vi "UHR-Fleezers Control (host) - 11.1.vi"() -> ()   [LabVIEW 2012] (continued)
        n2504 = local read "Pump 3 contents"() -> (→"Pump 3 cont disp":string)
      }
      event "Reset Trap Pos. FB": Value Change {
        n2505 = event-data() -> ()  [unwired: 7 out]
        n2506 = xnode "Read/Write Control"("FPGA VI Reference In"=w4152, "error in"=w4151, "Trap Pos. FB Reset"="Reset Trap Pos. FB") -> ()  [unwired: 2 out]
      }
      event "Rem fb disp offset": Value Change {
        n2507 = event-data() -> ()  [unwired: 7 out]
        n2508 = local write "Rem fb disp offset"(FALSE ("Rem fb disp offset")) -> ()
        n2509 = local read "Mean T1 Position (nm)"() -> (w4154:dbl)
        n2510 = local read "FB Trap Pos Offset"() -> (w4155:dbl)
        n2511 = Subtract(x=w4155, y=w4154) -> (x-y=w4153:dbl)
        n2512 = local write "FB Trap Pos Offset"(w4153) -> ()
      }
      event "Threshold (nm)": Value Change {
        n2513 = event-data() -> ()  [unwired: 7 out]
        n2514 = flat-sequence {
          tunnel: w4159 -> [w4167]
          tunnel: w4158 -> [w4166]
          tunnel: [w4160] -> w4157
          tunnel: w4157 -> [w4173]
          frame #0 {
            n2515 = xnode "Read/Write Control"("FPGA VI Reference In"=w4167, "error in"=w4166) -> ("FPGA VI Reference Out"=w4163:T19, "error out"=w4162:errorcluster, "FPGA TTrig Thresh"=w4164:i64)
            n2516 = local read "Threshold stored (nm)"() -> (w4172:dbl)
            n2517 = local read "Threshold (nm)"() -> (w4160:dbl)
            n2518 = local read "AOM X Cal (nm/MHz)"() -> (w4170:dbl)
            n2519 = Subtract(x=w4160, y=w4172) -> (x-y=w4171:dbl)
            n2520 = Divide(x=w4171, y=w4170) -> (x/y=w4168:dbl)
            n2521 = call "IR AOM freq to word.vi"("Frequency In (MHz)"=w4168) -> ("Frequency Word Out (double)"=w4169:dbl)
            n2522 = To Quad Integer(1:w4169) -> (0:w4165:i64)
            n2523 = Add(x=w4164, y=w4165) -> (x+y=w4161:i64)
            n2524 = xnode "Read/Write Control"("FPGA VI Reference In"=w4163, "error in"=w4162, "FPGA TTrig Thresh"=w4161) -> ()  [unwired: 2 out]
          }
          frame #1 {
            "Threshold stored (nm)" <- w4173
          }
        }
      }
      event "FB Trig Integrate": Value Change {
        n2525 = event-data() -> ()  [unwired: 7 out]
        n2526 = local read "FB Trig Integrate"() -> (w4175:u32)
        n2527 = xnode "Read/Write Control"("FPGA VI Reference In"=w4177, "error in"=w4176, "FB Trig Integrate"=w4175) -> ("error out"=w4174:errorcluster)  [unwired: 1 out]
      }
      event "11": Value Change {
        n2528 = event-data() -> ()  [unwired: 7 out]
        n2529 = local read "11"() -> (w4178:bool)
        n2530 = case shown="True" w4178 {
          frame False {
          }
          frame True {
            n2531 = local read "Messages"() -> (w4180:string)
            n2532 = call "Update messages.vi"("Message to add"="You kicked it up to 11!", "Old message string"=w4180) -> ("New message string"=w4181:string)
            n2533 = call <vilib>:"Beep.vi"() -> ()  [unwired: 12 in]
            n2534 = local write "Messages"(w4181) -> ()
          }
        }
      }
      event "Trap Pos. FB ON": Value Change {
        n2535 = event-data() -> ()  [unwired: 7 out]
        n2536 = xnode "Read/Write Control"("FPGA VI Reference In"=w4184, "error in"=w4183, "Force feedback"="Trap Pos. FB ON") -> ()  [unwired: 2 out]
      }
      event "Remove Action Offset": Value Change {
        n2537 = event-data() -> ()  [unwired: 7 out]
        n2538 = local write "Remove Action Offset"(FALSE ("Remove Action Offset")) -> ()
        n2539 = local read "Trap Pos. FB Mult Factor"() -> (w4189:i64)
        n2540 = local read "Trap Pos FB Action"() -> (w4187:i64)
        n2541 = local read "Trap Pos. FB Offset Factor"() -> (w4185:i64)
        n2542 = Multiply(x=w4189, y=w4187) -> (x*y=w4188:i64)
        n2543 = Add(x=w4188, y=w4185) -> (x+y=w4186:i64)
        n2544 = local write "Trap Pos. FB Offset Factor"(w4186) -> ()
        n2545 = xnode "Read/Write Control"("FPGA VI Reference In"=w4192, "error in"=w4191, "Trap Pos. FB Offset Factor"=w4186) -> ()  [unwired: 2 out]
      }
      event "Remove Unwinding Offset": Value Change {
        n2546 = event-data() -> ()  [unwired: 7 out]
        n2547 = local write "Remove Unwinding Offset"(FALSE ("Remove Action Offset")) -> ()
        n2548 = local read "Trap Pos. FB Mult Factor"() -> (w4204:i64)
        n2549 = local read "Trap Pos FB Action"() -> (w4202:i64)
        n2550 = local read "Trap Pos. FB Offset Factor"() -> (w4201:i64)
        n2551 = Multiply(x=w4204, y=w4202) -> (x*y=w4203:i64)
        n2552 = local read "Trap Pos. FB Mult Factor"() -> (w4200:i64)
        n2553 = Add(x=w4203, y=w4201) -> (x+y=w4194:i64)
        n2554 = Multiply(x=32768, y="factor") -> (x*y=w4197:dbl)
        n2555 = Multiply(x=w4197, y=w4200) -> (x*y=w4199:dbl)
        n2556 = Subtract(x=w4194, y=w4199) -> (x-y=w4198:dbl)
        n2557 = To Quad Integer(1:w4198) -> (0:w4193:i64)
        n2558 = xnode "Read/Write Control"("FPGA VI Reference In"=w4207, "error in"=w4206, "Trap Pos. FB Offset Factor"=w4193) -> ()  [unwired: 2 out]
        n2559 = local write "Trap Pos. FB Offset Factor"(w4193) -> ()
      }
      event "Trap Pos. FB Range", "Trap Pos. FB Gains", "Trap Pos. FB Mult Factor", "Trap Pos. FB Offset Factor", "Trap Pos FB Negate Action", "Trap Pos FB Monitor\nT1 or T2", "Differential FB?", "Negate Diff?": Value Change {
        n2560 = event-data() -> ()  [unwired: 7 out]
        n2561 = local read "Negate Diff?"() -> (w4208:bool)
        n2562 = xnode "Read/Write Control"("FPGA VI Reference In"=w4218, "error in"=w4217, "Trap Pos. FB Range"="Trap Pos. FB Range", "Trap Pos. FB Gains"="Trap Pos. FB Gains", "Trap Pos. FB Mult Factor"="Trap Pos. FB Mult Factor", "Trap Pos. FB Offset Factor"="Trap Pos. FB Offset Factor", "Trap Pos FB Negate Action"="Trap Pos FB Negate Action", "Trap Pos FB Monitor T1 or T2"="Trap Pos FB Monitor\nT1 or T2", "AI1 X Scale"="Trap Pos. AI1 X Pre-scale", "Negate Diff?"=w4208, "Diff FB Measurement?"="Differential FB?") -> ()  [unwired: 2 out]
      }
      event "Trap Pos FB SP", "Trap Pos FB SP 2", "Use SP 2": Value Change {
        n2563 = event-data() -> ()  [unwired: 7 out]
        n2564 = Select(t="Trap Pos FB SP 2", s="Use SP 2", f="Trap Pos FB SP") -> (s? t:f=w4219:fxp<+/-,16,1>)
        n2565 = xnode "Read/Write Control"("FPGA VI Reference In"=w4224, "error in"=w4223, "Trap Pos. FB SP"=w4219) -> ()  [unwired: 2 out]
      }
      event "Offset SP2 from SP1": Value Change {
        n2566 = event-data() -> ()  [unwired: 7 out]
        n2567 = local read "Trap Pos FB SP"() -> (w4227:fxp<+/-,16,1>)
        n2568 = Add(x=w4227, y="SP2 Offset") -> (x+y=w4225:fxp<+/-,16,1>)
        n2569 = property on="Trap Pos FB SP 2" class="DigNum (strict)"("Val(Sgnl)"=w4225) -> ()  [unwired: 2 in, 2 out]
        n2570 = local write "Offset SP2 from SP1"(FALSE ("Offset SP2 from SP1")) -> ()
      }
      event "Set Reading to\nSetpoint": Value Change {
        # "This is the actual PID input signal"
        n2571 = event-data() -> ()  [unwired: 7 out]
        n2572 = local write "Set Reading to\nSetpoint"(FALSE ("Set SP to Reading")) -> ()
        n2573 = xnode "Read/Write Control"("FPGA VI Reference In"=w4233, "error in"=w4232) -> ("FPGA VI Reference Out"=w4231:T19, "error out"=w4230:errorcluster, "Trap Pos FB Int-Norm Signal"=w4229:fxp<+/-,16,1>)
        n2574 = local read "Differential FB?"() -> (w4234:bool)
        n2575 = case shown="False" w4234 {
          tunnel: [w4239 w4246] -> w4236
          tunnel: w4229 -> [w4237 w4246]
          frame False {
            n2576 = local read "Trap Pos FB Monitor\nT1 or T2"() -> (w4242:bool)
            n2577 = local read "Trap X AI1 (DMA)"() -> (w4245:T13)
            n2578 = Unbundle By Name(w4245) -> ("Set 1"=w4244:fxp<+/-,16,1>, "Set 2"=w4243:fxp<+/-,16,1>)
            n2579 = Select(t=w4244, s=w4242, f=w4243) -> (s? t:f=w4241:fxp<+/-,16,1>)
            n2580 = Not(x="Set SP Using...") -> (.not. x?=w4238:bool)
            n2581 = Select(t=w4237, s=w4238, f=w4241) -> (s? t:f=w4239:fxp<+/-,16,1>)
          }
          frame True {
          }
        }
        n2582 = xnode "Read/Write Control"("FPGA VI Reference In"=w4231, "error in"=w4230, "Trap Pos. FB SP"=w4236) -> ()  [unwired: 2 out]
        n2583 = local write "Trap Pos FB SP"(w4236) -> ()
      }
      event "Trap Pos. FB Out Scale 2^n": Value Change {
        n2584 = event-data() -> ()  [unwired: 7 out]
        n2585 = Scale By Power Of 2(n="Trap Pos. FB Out Scale 2^n", x=ext 1.0) -> (x*2^n=w4247:ext)
        n2586 = property on="Trap Pos. FB Mult Factor" class="DigNum (strict)"("Val(Sgnl)"=w4247) -> ()  [unwired: 2 in, 2 out]
      }
      event "Trap Pos FB Int Count": Value Change {
        n2587 = event-data() -> ()  [unwired: 7 out]
        n2588 = xnode "Read/Write Control"("FPGA VI Reference In"=w4252, "error in"=w4251, "Trap Pos FB Int Count"="Trap Pos FB Int Count") -> ()  [unwired: 2 out]
      }
      event "Trap pos": Value Change {
        n2589 = event-data() -> ()  [unwired: 7 out]
        n2590 = case shown="True" "Trap pos" {
          frame False {
            n2591 = property on="Trap Delta Graph" class="WFGraph (strict)"("Visible"=TRUE) -> ()  [unwired: 2 in, 2 out]
            n2592 = property on="Saved trap pos" class="WFGraph (strict)"("Visible"=FALSE) -> ()  [unwired: 2 in, 2 out]
          }
          frame True {
            n2593 = property on="Saved trap pos" class="WFGraph (strict)"("Visible"=TRUE) -> ()  [unwired: 2 in, 2 out]
            n2594 = property on="Trap Delta Graph" class="WFGraph (strict)"("Visible"=FALSE) -> ()  [unwired: 2 in, 2 out]
          }
        }
      }
    }
    "error out 2" <- w3157
    n2595 = node-c288() -> ()  [unwired: 2 out]
  }
  n2596 = timed-loop "Oscillate Trap/AOM (fishing, debugging)" {
    tunnel: w6 -> [w4259]
    tunnel: [w4258] -> w100
    timing: w95 -> [_]
    timing-out: [_] -> w94
    stop <- w4258 stop-if-true
    n2597 = node-c288() -> ()  [unwired: 2 out]
    n2598 = event shown="[0] \"Oscillate Set 1\", \"Fish for Tether\": Value Change" {
      selector: _ -> [_ _ _]
      dyn-events: _ -> [_ _ _]
      timeout: _ -> [_ _ _]
      tunnel: w4259 -> [w4266 _ _]
      tunnel: [FALSE ("Stop All") _ w4855] -> w4258
      event "Oscillate Set 1", "Fish for Tether": Value Change {
        n2599 = event-data() -> ()  [unwired: 6 out]
        n2600 = local read "Oscillate Set 1"() -> (w4265:bool)
        n2601 = Or(x=w4265, y="Fish for Tether") -> (x .or. y?=w4263:bool)
        n2602 = case shown="True" w4263 {
          tunnel: w4266 -> [_ w4269]
          tunnel: "Fish for Tether" -> [_ w4268]
          frame False {
          }
          frame True {
            n2603 = case shown="True" w4268 {
              selector: w4268 -> [w4272 w4278]
              tunnel: [w4272 w4278] -> w4267
              frame False {
              }
              frame True {
                n2604 = local write "Scan axis 2"(TRUE) -> ()
                n2605 = local write "Tether"(FALSE ("Tether")) -> ()
                n2606 = local read "Flow ON during cal?"() -> (w4273:bool)
                n2607 = property on="Trap Delta (MHz)" class="DigNum (strict)"("Val(Sgnl)"="Furthest Delta (MHz)") -> ()  [unwired: 2 in, 2 out]
                n2608 = Or(x="Flow ON during \nfishing?", y=w4273) -> (x .or. y?=w4274:bool)
                n2609 = Wait (ms)(milliseconds to wait=u32 500) -> ()  [unwired: 1 out]
                n2610 = property on="Sample Channel\nFlow" class="Bool (strict)"("Val(Sgnl)"=w4274) -> ()  [unwired: 2 in, 2 out]
              }
            }
            n2611 = node-c288() -> (w4271:T21)  [unwired: 4 out]
            n2612 = timed-loop "Oscillate AOD" {
              timing: w4271 -> [_]
              timing-out: [_] -> w4270
              tunnel: w4269 -> [w4288]
              tunnel: w4267 -> [w4281]
              i -> [w4290]
              stop <- w4287 stop-if-true
              n2613 = node-c288() -> (w4289:i64)  [unwired: 1 out]
              n2614 = flat-sequence {
                tunnel: w4290 -> [w4317]
                tunnel: w4289 -> [w4316]
                tunnel: w4288 -> [w4295]
                tunnel: w4281 -> [w4298]
                tunnel: [w4298] -> w4286
                tunnel: [w4297] -> w4285
                tunnel: [w4294] -> w4284
                tunnel: [w4291] -> w4282
                tunnel: w4286 -> [w4353]
                tunnel: w4285 -> [w4351]
                tunnel: w4284 -> [w4350]
                tunnel: [w4349] -> w4283
                tunnel: w4282 -> [w4348]
                tunnel: [w4425] -> w4287
                tunnel: w4283 -> [w4424]
                frame #0 {
                  n2615 = Divide(x=w4316, y=i64 1000) -> (x/y=w4311:dbl)
                  n2616 = Multiply(x=w4311, y=w4317) -> (x*y=w4313:dbl)
                  n2617 = local read "BD 1 Frequency 2 (MHz)"() -> (w4296:dbl)
                  n2618 = Multiply(x="Osc. freq. (Hz)", y=6.283185307179586) -> (x*y=w4314:dbl)
                  n2619 = Multiply(x=w4314, y=w4313) -> (x*y=w4293:dbl)
                  n2620 = local read "BD 1 Frequency 1 (MHz)"() -> (w4301:dbl)
                  n2621 = local read "BD 2 Frequency 1 (MHz)"() -> (w4300:dbl)
                  n2622 = case shown="True" w4298 {
                    tunnel: w4293 -> [w4323 w4328]
                    tunnel: w4301 -> [_ w4339]
                    tunnel: w4296 -> [_ w4340]
                    tunnel: [w4320 w4334] -> w4299
                    tunnel: [FALSE w4331] -> w4294
                    tunnel: [0.0 w4324] -> w4291
                    frame False {
                      n2623 = Sine(x=w4323) -> (sin(x)=w4321:dbl)
                      n2624 = Multiply(x=w4321, y="Osc. amp. (MHz)") -> (x*y=w4320:dbl)
                    }
                    frame True {
                      n2625 = Cosine(x=w4328) -> (cos(x)=w4343:dbl)
                      n2626 = Subtract(x=w4340, y=w4339) -> (x-y=w4338:dbl)
                      n2627 = Decrement(x=w4343) -> (x-1=w4342:dbl)
                      n2628 = Subtract(x=w4338, y="Closest Delta (MHz)") -> (x-y=w4335:dbl)
                      n2629 = Divide(x=w4342, y=-2.0) -> (x/y=w4336:dbl)
                      n2630 = Multiply(x=w4336, y=w4335) -> (x*y=w4334:dbl)
                      n2631 = local read "Vec Mean of T1 T2"() -> (w4330:dbl[])
                      n2632 = Greater?(x=w4330, y="Stop F (pN)") -> (0:w4332:bool[])
                      n2633 = Or Array Elements(Boolean array=w4332) -> (logical OR=w4331:bool)
                      n2634 = Divide(x=w4328, y=6.283185307179586) -> (x/y=w4327:dbl)
                      n2635 = Round Toward +Infinity(x=w4327) -> (ceil(x): smallest int >= x=w4324:dbl)
                      "Attempts" <- w4324
                      n2636 = Greater?(x=w4324, y="Attempt Limit") -> (0:w4326:bool)
                      n2637 = case shown="True" w4326 {
                        frame False {
                        }
                        frame True {
                          n2638 = local write "Fish for Tether"(FALSE ("Fish for Tether")) -> ()
                          n2639 = call <vilib>:"Beep.vi"() -> ()  [unwired: 3 in, 9 out]
                          n2640 = local read "Messages"() -> (w4345:string)
                          n2641 = call "Update messages.vi"("Message to add"="Tether fishing timeout." ("Messages"), "Old message string"=w4345) -> ("New message string"=→"Messages":string)
                        }
                      }
                    }
                  }
                  n2642 = Select(t=w4301, s="Scan axis 2", f=w4300) -> (s? t:f=w4304:dbl)
                  n2643 = Add(x=w4299, y=w4304) -> (x+y=w4297:dbl)
                  n2644 = Select(t=w4297, s="Scan axis 2", f=w4301) -> (s? t:f=w4307:dbl)
                  n2645 = Select(t=w4300, s="Scan axis 2", f=w4297) -> (s? t:f=w4306:dbl)
                  n2646 = local read "Y RF Frequency Limits (MHz)"() -> (w4302:T16)
                  n2647 = local read "X RF Frequency Limits (MHz)"() -> (w4303:T16)
                  n2648 = local read "BD 1 Frequency 3 (MHz)"() -> (w4310:dbl)
                  n2649 = local read "BD 2 Frequency 2 (MHz)"() -> (w4309:dbl)
                  n2650 = local read "BD 2 Frequency 3 (MHz)"() -> (w4308:dbl)
                  n2651 = call "set RF board frequency - interlace.vi"("Board 2 Frequency Limits"=w4302, "Board 1 Frequency Limits"=w4303, "FPGA VI Reference In"=w4295, "Board 2 Frequency 3 (MHz)"=w4308, "Board 1 Frequency 3 (MHz)"=w4310, "Board 2 Frequency 2 (MHz)"=w4309, "Board 2 Frequency 1 (MHz)"=w4306, "Board 1 Frequency 2 (MHz)"=w4296, "Board 1 Frequency 1  (MHz)"=w4307) -> ()  [unwired: 1 in, 2 out]
                }
                frame #1 {
                  n2652 = And(x=w4353, y=w4350) -> (x .and. y?=w4352:bool)
                  n2653 = case "Only if were fishing and now formed tether" shown="False" w4352 {
                    tunnel: w4351 -> [w4355 w4370]
                    tunnel: [w4354 w4369] -> w4349
                    tunnel: w4348 -> [_ w4365]
                    frame False {
                      n2654 = local read "Fish for Tether"() -> (w4354:bool)
                      n2655 = case shown="False" w4354 {
                        tunnel: w4355 -> [w4356 _]
                        frame False {
                          n2656 = property on="BD 1 Frequency 1 (MHz)" class="DigNum (strict)"("Val(Sgnl)"=w4356) -> ()  [unwired: 2 in, 2 out]
                        }
                        frame True {
                        }
                      }
                    }
                    frame True {
                      w4369 = FALSE ("Fish for Tether")
                      n2657 = call <vilib>:"Beep.vi"() -> ()  [unwired: 3 in, 9 out]
                      n2658 = Number To Decimal String(number=w4365, width (-)=i16 1) -> (decimal integer string=w4363:string)
                      n2659 = Concatenate Strings("Formed tether in ", w4363, " attempt(s)." ("string")) -> (w4360:string)
                      n2660 = local read "Messages"() -> (w4367:string)
                      n2661 = local write "Fish for Tether"(w4369) -> ()
                      n2662 = call "Update messages.vi"("Message to add"=w4360, "Old message string"=w4367) -> ("New message string"=w4366:string)
                      n2663 = local write "Messages"(w4366) -> ()
                      n2664 = Get Date/Time In Seconds() -> (seconds since 1Jan1904=→"Time tether formed":timestamp)
                      n2665 = local read "Flow ON during cal?"() -> (w4357:bool)
                      n2666 = property on="Sample Channel\nFlow" class="Bool (strict)"("Val(Sgnl)"=w4357) -> (error out=w4358:errorcluster)  [unwired: 2 in, 1 out]
                      n2667 = case shown="\"2\", \"3\", \"4\", \"5\", \"6\"" "Then..." {
                        selector: "Then..." -> [_ w4373]
                        tunnel: w4370 -> [w4372 _]
                        tunnel: w4358 -> [_ _]
                        frame "1", Default {
                          n2668 = property on="BD 1 Frequency 1 (MHz)" class="DigNum (strict)"("Val(Sgnl)"=w4372) -> ()  [unwired: 2 in, 2 out]
                        }
                        frame "2", "3", "4", "5", "6" {
                          n2669 = flat-sequence {
                            tunnel: w4373 -> [w4375]
                            frame #0 {
                              n2670 = property on="Trap Delta (MHz)" class="DigNum (strict)"("Val(Sgnl)"="Move to Delta 1 (MHz)") -> ()  [unwired: 2 in, 2 out]
                            }
                            frame #1 {
                              n2671 = case shown="\"5\", \"6\"" w4375 {
                                selector: w4375 -> [w4378 w4388 _]
                                frame "3", "4" {
                                n2672 = flat-sequence {
                                tunnel: w4378 -> [w4379]
                                tunnel: [w4379] -> w4376
                                tunnel: [w4381] -> w4377
                                tunnel: w4376 -> [w4381]
                                tunnel: w4377 -> [w4385]
                                frame #0 {
                                n2673 = property on="Green Laser ON/Interlacing" class="Bool (strict)"("Val(Sgnl)"=TRUE ("Value (Signaling)")) -> ()  [unwired: 2 in, 2 out]
                                }
                                frame #1 {
                                n2674 = Multiply(x="Wait Before Save (s)", y=u32 1000 ("x")) -> (x*y=w4383:u32)
                                n2675 = Wait (ms)(milliseconds to wait=w4383) -> ()  [unwired: 1 out]
                                }
                                frame #2 {
                                n2676 = property on="Start Saving" class="Bool (strict)"("Value"=TRUE ("Start Saving")) -> ()  [unwired: 2 in, 2 out]
                                n2677 = case shown="\"4\"" w4385 {
                                frame Default {
                                }
                                frame "4" {
                                n2678 = property on="Fl. Triggered..." class="Bool (strict)"("Val(Sgnl)"=TRUE ("Value (Signaling)")) -> ()  [unwired: 2 in, 2 out]
                                }
                                }
                                }
                                }
                                }
                                frame "5", "6" {
                                n2679 = stacked-sequence {
                                tunnel: w4388 -> [_ _ _ _ _ _ w4400]
                                frame #0 {
                                n2680 = Replace Array Subset(array=u32[] [0] ("Index Values"), new element="Raster Set Upon Tether", index=0) -> (w4389:u32[])
                                n2681 = property on="Saved AOD Raster Scan Parameter Sets" class="Arr (strict)"("Index Values"=w4389) -> ()  [unwired: 2 in, 2 out]
                                }
                                frame #1 {
                                n2682 = Wait (ms)(milliseconds to wait=u32 500) -> ()  [unwired: 1 out]
                                }
                                frame #2 {
                                n2683 = property on="Load parameters" class="Bool (strict)"("Val(Sgnl)"=TRUE ("Value (Signaling)")) -> ()  [unwired: 2 in, 2 out]
                                n2684 = case shown="True" "Green ON During Raster" {
                                frame False {
                                }
                                frame True {
                                n2685 = property on="Green Laser ON/Interlacing" class="Bool (strict)"("Val(Sgnl)"=TRUE ("Value (Signaling)")) -> ()  [unwired: 2 in, 2 out]
                                }
                                }
                                }
                                frame #3 {
                                n2686 = Wait (ms)(milliseconds to wait=u32 500) -> ()  [unwired: 1 out]
                                }
                                frame #4 {
                                n2687 = property on="Trap Raster Scan" class="Bool (strict)"("Val(Sgnl)"=TRUE ("Value (Signaling)")) -> ()  [unwired: 2 in, 2 out]
                                }
                                frame #5 {
                                n2688 = Wait (ms)(milliseconds to wait=u32 2000) -> ()  [unwired: 1 out]
                                }
                                frame #6 {
                                n2689 = flat-sequence {
                                tunnel: w4400 -> [w4407]
                                frame #0 {
                                n2690 = while {
                                stop <- w4403 stop-if-true
                                n2691 = local read "Raster Scanning..."() -> (w4402:bool)
                                n2692 = local read "Saving..."() -> (w4405:bool)
                                n2693 = Wait (ms)(milliseconds to wait=u32 100) -> ()  [unwired: 1 out]
                                n2694 = Not(x=w4405) -> (.not. x?=w4404:bool)
                                n2695 = Not(x=w4402) -> (.not. x?=w4401:bool)
                                n2696 = And(x=w4404, y=w4401) -> (x .and. y?=w4403:bool)
                                }
                                }
                                frame #1 {
                                n2697 = local read "Tether"() -> (w4408:bool)
                                n2698 = case shown="True" w4408 {
                                tunnel: w4407 -> [_ w4410]
                                frame False {
                                n2699 = property on="Fish for Tether" class="Bool (strict)"("Val(Sgnl)"="Fish again after \nraster break?") -> ()  [unwired: 2 in, 2 out]
                                }
                                frame True {
                                n2700 = stacked-sequence {
                                tunnel: w4410 -> [_ w4414 _ _]
                                frame #0 {
                                n2701 = property on="Trap Delta (MHz)" class="DigNum (strict)"("Val(Sgnl)"="Move to Delta 2 (MHz)") -> ()  [unwired: 2 in, 2 out]
                                n2702 = case shown="True" "Flow ON after\ntether testing?" {
                                frame False {
                                }
                                frame True {
                                n2703 = property on="Sample Channel\nFlow" class="Bool (strict)"("Val(Sgnl)"=TRUE ("Value (Signaling)")) -> ()  [unwired: 2 in, 2 out]
                                }
                                }
                                }
                                frame #1 {
                                n2704 = flat-sequence {
                                tunnel: w4414 -> [w4416]
                                frame #0 {
                                n2705 = Wait (ms)(milliseconds to wait=u32 500) -> ()  [unwired: 1 out]
                                }
                                frame #1 {
                                n2706 = case shown="\"6\"" w4416 {
                                frame Default {
                                }
                                frame "6" {
                                n2707 = property on="Green Laser ON/Interlacing" class="Bool (strict)"("Val(Sgnl)"=TRUE ("Green Laser ON/Interlacing")) -> ()  [unwired: 2 in, 2 out]
                                }
                                }
                                }
                                frame #2 {
                                n2708 = Wait (ms)(milliseconds to wait=u32 500) -> ()  [unwired: 1 out]
                                }
                                frame #3 {
                                n2709 = local write "Start Saving"("Save at end (5, 6)") -> ()
                                }
                                }
                                }
                                frame #2 {
                                n2710 = local read "Bead Sep. Int. Time (s)"() -> (w4422:dbl)
                                n2711 = Multiply(x=w4422, y=1000.0) -> (x*y=w4421:dbl)
                                n2712 = Wait (ms)(milliseconds to wait=w4421) -> ()  [unwired: 1 out]
                                }
                                frame #3 {
                                n2713 = property on="Remove Offset" class="Bool (strict)"("Val(Sgnl)"=TRUE ("Value (Signaling)")) -> ()  [unwired: 2 in, 2 out]
                                }
                                }
                                }
                                }
                                }
                                }
                                }
                                }
                                }
                                frame "2", Default {
                                }
                              }
                            }
                          }
                        }
                      }
                      "Tether" <- "Tether Alarm?"
                    }
                  }
                }
                frame #2 {
                  n2714 = local read "Oscillate Set 1"() -> (w4429:bool)
                  n2715 = local read "Stop All"() -> (w4427:bool)
                  n2716 = Or(x=w4429, y=w4424) -> (x .or. y?=w4426:bool)
                  n2717 = Not(x=w4426) -> (.not. x?=w4428:bool)
                  n2718 = Compound Arithmetic op=OR(w4427, w4428) -> (w4425:bool)
                }
              }
              n2719 = node-c288() -> ()  [unwired: 2 out]
            }
            n2720 = node-c288(w4270) -> ()  [unwired: 1 out]
          }
        }
      }
      event "Fl. Triggered...": Value Change {
        n2721 = event-data() -> ()  [unwired: 7 out]
        n2722 = case shown="True" "Fl. Triggered..." {
          frame False {
          }
          frame True {
            n2723 = node-c288() -> (w4440:T21)  [unwired: 4 out]
            n2724 = timed-loop {
              timing: w4440 -> [_]
              timing-out: [_] -> w4439
              tunnel: "Action" -> [w4448]
              shift-right: [w4445] -> _
              shift-left: u8 255 -> [w4447]
              shift-right: [w4442] -> _
              shift-left: 255 -> [w4444]
              stop <- w4441 stop-if-true
              # "Reset confocal spot"
              n2725 = node-c288() -> ()  [unwired: 2 out]
              n2726 = flat-sequence {
                tunnel: w4448 -> [w4468]
                tunnel: w4447 -> [w4467]
                tunnel: [w4466] -> w4446
                tunnel: w4444 -> [w4453]
                tunnel: [w4452] -> w4443
                tunnel: [w4847] -> w4441
                tunnel: w4446 -> [w4846]
                tunnel: [w4846] -> w4445
                tunnel: [w4845] -> w4442
                tunnel: w4443 -> [w4845]
                frame #0 {
                  n2727 = local read "Delta Fl. 2"() -> (w4465:dbl)
                  n2728 = local read "Delta Fl. 1"() -> (w4460:dbl)
                  n2729 = Multiply(x="Fl. Delta Thresh. (kHz)", y=1000.0) -> (x*y=w4455:dbl)
                  n2730 = Select(t=w4460, s="APD to Watch", f=w4465) -> (s? t:f=w4456:dbl)
                  n2731 = Greater?(x=w4456, y=w4455) -> (0:w4461:bool)
                  n2732 = Or(x="Force Yank", y=w4461) -> (x .or. y?=w4459:bool)
                  n2733 = And(x=w4459, y="Yank when?") -> (x .and. y?=w4457:bool)
                  n2734 = case shown="False" w4457 {
                    tunnel: w4468 -> [w4471 w4672]
                    tunnel: w4467 -> [w4473 w4668]
                    tunnel: [w4473 w4666] -> w4466
                    tunnel: w4456 -> [w4479 _]
                    tunnel: w4455 -> [w4478 _]
                    tunnel: "Force Yank" -> [w4476 _]
                    tunnel: w4453 -> [w4475 w4665]
                    tunnel: [w4474 w4665] -> w4452
                    frame False {
                      n2735 = Negate(x=w4478) -> (-x=w4470:dbl)
                      n2736 = local write "Fl. High"(TRUE ("Fl. High")) -> ()
                      n2737 = Less?(x=w4479, y=w4470) -> (x < y?=w4477:bool)
                      n2738 = Or(x=w4476, y=w4477) -> (x .or. y?=w4472:bool)
                      n2739 = case shown="True" w4472 {
                        tunnel: w4475 -> [w4480 w4490]
                        tunnel: [w4480 w4489] -> w4474
                        tunnel: w4471 -> [_ w4488]
                        frame False {
                        }
                        frame True {
                          n2740 = flat-sequence {
                            tunnel: w4490 -> [w4496]
                            tunnel: w4488 -> [w4493]
                            tunnel: [w4495] -> w4487
                            tunnel: [w4494] -> w4486
                            tunnel: [w4493] -> w4485
                            tunnel: w4484 -> [w4492]
                            tunnel: [w4492] -> w4483
                            tunnel: w4482 -> [w4491]
                            tunnel: [w4491] -> w4481
                            tunnel: [w4567] -> w4489
                            tunnel: w4487 -> [w4567]
                            tunnel: w4486 -> [w4566]
                            tunnel: w4485 -> [w4565]
                            tunnel: w4483 -> [w4564]
                            tunnel: w4481 -> [w4563]
                            frame #0 {
                              n2741 = call <vilib>:"Beep.vi"() -> ()  [unwired: 12 in]
                              n2742 = local write "Waiting"(FALSE ("Waiting")) -> ()
                              n2743 = Increment(x=w4496) -> (x+1=w4495:i32)
                              n2744 = case shown="\"Yank\"" w4493 {
                                tunnel: w4495 -> [_ w4501 _]
                                frame "Alarm", Default {
                                }
                                frame "Yank" {
                                n2745 = flat-sequence {
                                tunnel: w4501 -> [w4504]
                                tunnel: [w4503] -> w4500
                                tunnel: [w4502] -> w4499
                                tunnel: w4500 -> [w4514]
                                tunnel: w4499 -> [w4515]
                                frame #0 {
                                n2746 = local read "Yank Delay (s)"() -> (w4507:dbl)
                                n2747 = local read "N Array El"() -> (w4502:u8)
                                n2748 = Quotient & Remainder(x=w4504, y=w4502) -> (x-y*floor(x/y)=w4503:i32)  [unwired: 1 out]
                                n2749 = Multiply(x=w4507, y=1000.0) -> (x*y=w4505:dbl)
                                n2750 = Wait (ms)(milliseconds to wait=w4505) -> ()  [unwired: 1 out]
                                }
                                frame #1 {
                                n2751 = local read "Yank to which?"() -> (w4509:bool)
                                n2752 = local read "Random Choice"() -> (w4519:bool)
                                n2753 = local read "Yank to Trap Delta (MHz)"() -> (w4512:dbl[])
                                n2754 = local read "Yank to SP"() -> (w4513:dbl[])
                                n2755 = Random Number (0-1)() -> (number: 0 to 1=w4518:dbl)
                                n2756 = Multiply(x=w4515, y=w4518) -> (x*y=w4517:dbl)
                                n2757 = Round Toward -Infinity(1:w4517) -> (0:w4516:dbl)
                                n2758 = Select(t=w4516, s=w4519, f=w4514) -> (s? t:f=w4510:dbl)
                                n2759 = Select(t=w4512, s=w4509, f=w4513) -> (s? t:f=w4511:dbl[])
                                n2760 = Index Array(array=w4511, index=w4510) -> (element=w4508:dbl)
                                n2761 = case shown="True" w4509 {
                                tunnel: w4508 -> [w4520 w4547]
                                frame False {
                                n2762 = flat-sequence {
                                tunnel: w4520 -> [w4521]
                                frame #0 {
                                n2763 = property on="Trap Pos FB SP" class="DigNum (strict)"("Val(Sgnl)"=w4521) -> ()  [unwired: 2 in, 2 out]
                                }
                                frame #1 {
                                n2764 = Wait (ms)(milliseconds to wait=u32 700) -> ()  [unwired: 1 out]
                                }
                                frame #2 {
                                n2765 = local read "Action (%)"() -> (w4526:dbl)
                                n2766 = Absolute Value(x=w4526) -> (abs(x)=w4525:dbl)
                                n2767 = Greater?(x=w4525, y=70.0) -> (0:w4523:bool)
                                n2768 = property on="Remove Action Offset" class="Bool (strict)"("Val(Sgnl)"=w4523) -> ()  [unwired: 2 in, 2 out]
                                }
                                frame #3 {
                                n2769 = for {
                                N: 4 -> [_]
                                n2770 = flat-sequence {
                                frame #0 {
                                n2771 = Wait (ms)(milliseconds to wait=u32 500) -> ()  [unwired: 1 out]
                                }
                                frame #1 {
                                n2772 = local read "Action (%)"() -> (w4532:dbl)
                                n2773 = Absolute Value(x=w4532) -> (abs(x)=w4531:dbl)
                                n2774 = Greater?(x=w4531, y=70.0) -> (0:w4529:bool)
                                n2775 = property on="Remove Action Offset" class="Bool (strict)"("Val(Sgnl)"=w4529) -> ()  [unwired: 2 in, 2 out]
                                }
                                }
                                }
                                }
                                frame #4 {
                                n2776 = Wait (ms)(milliseconds to wait=u32 500) -> ()  [unwired: 1 out]
                                }
                                frame #5 {
                                n2777 = local read "Mean"() -> (w4540:dbl)
                                n2778 = Greater?(x=w4540, y=11.0) -> (0:w4534:bool)
                                n2779 = Not(x=w4534) -> (.not. x?=w4535:bool)
                                n2780 = And(x=w4535, y="Shift confocal") -> (x .and. y?=w4537:bool)
                                n2781 = And(x=w4534, y="Shift confocal") -> (x .and. y?=w4538:bool)
                                n2782 = case shown="True" w4538 {
                                frame False {
                                }
                                frame True {
                                n2783 = local read "Confocal Y 2 (V)"() -> (w4544:dbl)
                                n2784 = local read "Confocal X 2 (V)"() -> (w4543:dbl)
                                n2785 = property on="AO1" class="Slide (strict)"("Val(Sgnl)"=w4544) -> ()  [unwired: 2 in, 2 out]
                                n2786 = property on="AO2" class="Slide (strict)"("Val(Sgnl)"=w4543) -> ()  [unwired: 2 in, 2 out]
                                }
                                }
                                n2787 = case shown="True" w4537 {
                                frame False {
                                }
                                frame True {
                                n2788 = local read "Confocal Y 1 (V)"() -> (w4542:dbl)
                                n2789 = local read "Confocal X 1 (V)"() -> (w4541:dbl)
                                n2790 = property on="AO1" class="Slide (strict)"("Val(Sgnl)"=w4542) -> ()  [unwired: 2 in, 2 out]
                                n2791 = property on="AO2" class="Slide (strict)"("Val(Sgnl)"=w4541) -> ()  [unwired: 2 in, 2 out]
                                }
                                }
                                }
                                frame #6 {
                                n2792 = Wait (ms)(milliseconds to wait=u32 1500) -> ()  [unwired: 1 out]
                                }
                                frame #7 {
                                n2793 = property on="Rem fb disp offset" class="Bool (strict)"("Val(Sgnl)"=TRUE ("Value (Signaling)")) -> ()  [unwired: 2 in, 2 out]
                                }
                                }
                                }
                                frame True {
                                n2794 = flat-sequence {
                                tunnel: w4547 -> [w4548]
                                frame #0 {
                                n2795 = property on="Trap Delta (MHz)" class="DigNum (strict)"("Val(Sgnl)"=w4548) -> ()  [unwired: 2 in, 2 out]
                                }
                                frame #1 {
                                n2796 = Wait (ms)(milliseconds to wait=u32 500) -> ()  [unwired: 1 out]
                                }
                                frame #2 {
                                n2797 = local read "Shift confocal"() -> (w4554:bool)
                                n2798 = local read "Mean"() -> (w4556:dbl)
                                n2799 = Greater?(x=w4556, y=11.0) -> (0:w4553:bool)
                                n2800 = Not(x=w4553) -> (.not. x?=w4552:bool)
                                n2801 = And(x=w4552, y=w4554) -> (x .and. y?=w4550:bool)
                                n2802 = And(x=w4553, y=w4554) -> (x .and. y?=w4551:bool)
                                n2803 = case shown="True" w4551 {
                                frame False {
                                }
                                frame True {
                                n2804 = local read "Confocal Y 2 (V)"() -> (w4560:dbl)
                                n2805 = local read "Confocal X 2 (V)"() -> (w4559:dbl)
                                n2806 = property on="AO2" class="Slide (strict)"("Val(Sgnl)"=w4559) -> ()  [unwired: 2 in, 2 out]
                                n2807 = property on="AO1" class="Slide (strict)"("Val(Sgnl)"=w4560) -> ()  [unwired: 2 in, 2 out]
                                }
                                }
                                n2808 = case shown="True" w4550 {
                                frame False {
                                }
                                frame True {
                                n2809 = local read "Confocal X 1 (V)"() -> (w4557:dbl)
                                n2810 = local read "Confocal Y 1 (V)"() -> (w4558:dbl)
                                n2811 = property on="AO2" class="Slide (strict)"("Val(Sgnl)"=w4557) -> ()  [unwired: 2 in, 2 out]
                                n2812 = property on="AO1" class="Slide (strict)"("Val(Sgnl)"=w4558) -> ()  [unwired: 2 in, 2 out]
                                }
                                }
                                }
                                }
                                }
                                }
                                }
                                }
                                }
                                frame "Image" {
                                n2813 = property on="Confocal Image" class="Bool (strict)"("Val(Sgnl)"=TRUE ("Value (Signaling)")) -> ()  [unwired: 2 in, 2 out]
                                }
                              }
                              n2814 = local write "Fl. High"(FALSE ("Fl. High")) -> ()
                              n2815 = local read "Time (s)"() -> (w4494:dbl)
                            }
                            frame #1 {
                              n2816 = case shown="True" "Auto F Reset" {
                                tunnel: w4566 -> [_ w4571]
                                tunnel: w4565 -> [_ w4570]
                                tunnel: w4564 -> [_ w4569]
                                tunnel: w4563 -> [_ w4568]
                                frame False {
                                }
                                frame True {
                                n2817 = node-c288() -> (w4573:T21)  [unwired: 4 in]
                                n2818 = timed-loop {
                                timing: w4573 -> [_]
                                timing-out: [_] -> w4572
                                tunnel: w4571 -> [w4578]
                                tunnel: w4570 -> [w4577]
                                tunnel: w4569 -> [w4576]
                                tunnel: w4568 -> [w4575]
                                stop <- w4574 stop-if-true
                                n2819 = node-c288() -> ()  [unwired: 1 in, 1 out]
                                n2820 = local read "Fl. Delta Thresh. (kHz)"() -> (w4587:dbl)
                                n2821 = local read "APD to Watch"() -> (w4588:bool)
                                n2822 = local read "Delta Fl. 1"() -> (w4589:dbl)
                                n2823 = local read "Delta Fl. 2"() -> (w4590:dbl)
                                n2824 = local read "Fl. Triggered..."() -> (w4581:bool)
                                n2825 = local read "Stop All"() -> (w4582:bool)
                                n2826 = local read "Reset Force"() -> (w4580:bool)
                                n2827 = Multiply(x=w4587, y=1000.0) -> (x*y=w4585:dbl)
                                n2828 = Not(x=w4581) -> (.not. x?=w4579:bool)
                                n2829 = Select(t=w4589, s=w4588, f=w4590) -> (s? t:f=w4584:dbl)
                                n2830 = Greater?(x=w4584, y=w4585) -> (0:w4583:bool)
                                n2831 = Compound Arithmetic op=OR(w4583, w4582, w4579, w4580) -> (w4574:bool)
                                n2832 = case shown="True" w4574 {
                                tunnel: w4578 -> [_ w4594]
                                tunnel: w4577 -> [_ w4598]
                                tunnel: w4576 -> [_ w4597]
                                tunnel: w4575 -> [_ w4596]
                                frame False {
                                }
                                frame True {
                                n2833 = case shown="\"Yank\"" w4598 {
                                tunnel: w4597 -> [_ w4608]
                                tunnel: w4596 -> [_ w4606]
                                frame "Image", Default {
                                }
                                frame "Yank" {
                                n2834 = flat-sequence {
                                tunnel: [w4611] -> w4609
                                tunnel: w4608 -> [w4611]
                                tunnel: [w4610] -> w4607
                                tunnel: w4606 -> [w4610]
                                tunnel: w4609 -> [w4617]
                                tunnel: w4607 -> [w4615]
                                frame #0 {
                                n2835 = local read "Yank Delay (s)"() -> (w4614:dbl)
                                n2836 = Multiply(x=w4614, y=1000.0) -> (x*y=w4612:dbl)
                                n2837 = Wait (ms)(milliseconds to wait=w4612) -> ()  [unwired: 1 out]
                                }
                                frame #1 {
                                n2838 = local read "Yank to which?"() -> (w4616:bool)
                                n2839 = case shown="False" w4616 {
                                tunnel: w4617 -> [_ w4645]
                                tunnel: w4615 -> [w4618 _]
                                frame False {
                                n2840 = flat-sequence {
                                tunnel: w4618 -> [w4619]
                                frame #0 {
                                n2841 = property on="Trap Pos FB SP" class="DigNum (strict)"("Val(Sgnl)"=w4619) -> ()  [unwired: 2 in, 2 out]
                                }
                                frame #1 {
                                n2842 = Wait (ms)(milliseconds to wait=u32 700) -> ()  [unwired: 1 out]
                                }
                                frame #2 {
                                n2843 = local read "Action (%)"() -> (w4624:dbl)
                                n2844 = Absolute Value(x=w4624) -> (abs(x)=w4623:dbl)
                                n2845 = Greater?(x=w4623, y=70.0) -> (0:w4621:bool)
                                n2846 = property on="Remove Action Offset" class="Bool (strict)"("Val(Sgnl)"=w4621) -> ()  [unwired: 2 in, 2 out]
                                }
                                frame #3 {
                                n2847 = for {
                                N: 4 -> [_]
                                n2848 = flat-sequence {
                                frame #0 {
                                n2849 = Wait (ms)(milliseconds to wait=u32 500) -> ()  [unwired: 1 out]
                                }
                                frame #1 {
                                n2850 = local read "Action (%)"() -> (w4630:dbl)
                                n2851 = Absolute Value(x=w4630) -> (abs(x)=w4629:dbl)
                                n2852 = Greater?(x=w4629, y=70.0) -> (0:w4627:bool)
                                n2853 = property on="Remove Action Offset" class="Bool (strict)"("Val(Sgnl)"=w4627) -> ()  [unwired: 2 in, 2 out]
                                }
                                }
                                }
                                }
                                frame #4 {
                                n2854 = Wait (ms)(milliseconds to wait=u32 500) -> ()  [unwired: 1 out]
                                }
                                frame #5 {
                                n2855 = local read "Shift confocal"() -> (w4635:bool)
                                n2856 = local read "Mean"() -> (w4638:dbl)
                                n2857 = Greater?(x=w4638, y=11.0) -> (0:w4634:bool)
                                n2858 = Not(x=w4634) -> (.not. x?=w4633:bool)
                                n2859 = And(x=w4634, y=w4635) -> (x .and. y?=w4636:bool)
                                n2860 = And(x=w4633, y=w4635) -> (x .and. y?=w4632:bool)
                                n2861 = case shown="True" w4636 {
                                frame False {
                                }
                                frame True {
                                n2862 = local read "Confocal X 2 (V)"() -> (w4641:dbl)
                                n2863 = local read "Confocal Y 2 (V)"() -> (w4642:dbl)
                                n2864 = property on="AO2" class="Slide (strict)"("Val(Sgnl)"=w4641) -> ()  [unwired: 2 in, 2 out]
                                n2865 = property on="AO1" class="Slide (strict)"("Val(Sgnl)"=w4642) -> ()  [unwired: 2 in, 2 out]
                                }
                                }
                                n2866 = case shown="True" w4632 {
                                frame False {
                                }
                                frame True {
                                n2867 = local read "Confocal Y 1 (V)"() -> (w4640:dbl)
                                n2868 = local read "Confocal X 1 (V)"() -> (w4639:dbl)
                                n2869 = property on="AO1" class="Slide (strict)"("Val(Sgnl)"=w4640) -> ()  [unwired: 2 in, 2 out]
                                n2870 = property on="AO2" class="Slide (strict)"("Val(Sgnl)"=w4639) -> ()  [unwired: 2 in, 2 out]
                                }
                                }
                                }
                                frame #6 {
                                n2871 = Wait (ms)(milliseconds to wait=u32 1500) -> ()  [unwired: 1 out]
                                }
                                frame #7 {
                                n2872 = property on="Rem fb disp offset" class="Bool (strict)"("Val(Sgnl)"=TRUE ("Value (Signaling)")) -> ()  [unwired: 2 in, 2 out]
                                }
                                }
                                }
                                frame True {
                                n2873 = flat-sequence {
                                tunnel: w4645 -> [w4646]
                                frame #0 {
                                n2874 = property on="Trap Delta (MHz)" class="DigNum (strict)"("Val(Sgnl)"=w4646) -> ()  [unwired: 2 in, 2 out]
                                }
                                frame #1 {
                                n2875 = Wait (ms)(milliseconds to wait=u32 500) -> ()  [unwired: 1 out]
                                }
                                frame #2 {
                                n2876 = local read "Shift confocal"() -> (w4652:bool)
                                n2877 = local read "Mean"() -> (w4653:dbl)
                                n2878 = Greater?(x=w4653, y=11.0) -> (0:w4651:bool)
                                n2879 = And(x=w4651, y=w4652) -> (x .and. y?=w4649:bool)
                                n2880 = Not(x=w4651) -> (.not. x?=w4650:bool)
                                n2881 = And(x=w4650, y=w4652) -> (x .and. y?=w4648:bool)
                                n2882 = case shown="True" w4649 {
                                frame False {
                                }
                                frame True {
                                n2883 = local read "Confocal Y 2 (V)"() -> (w4658:dbl)
                                n2884 = local read "Confocal X 2 (V)"() -> (w4657:dbl)
                                n2885 = property on="AO1" class="Slide (strict)"("Val(Sgnl)"=w4658) -> ()  [unwired: 2 in, 2 out]
                                n2886 = property on="AO2" class="Slide (strict)"("Val(Sgnl)"=w4657) -> ()  [unwired: 2 in, 2 out]
                                }
                                }
                                n2887 = case shown="True" w4648 {
                                frame False {
                                }
